vi "Load_Class_data.vi"() -> (2 "Classes":string[](array[string]), 3 "Styles and IDs":string[][](array[string]))   [LabVIEW 2025]
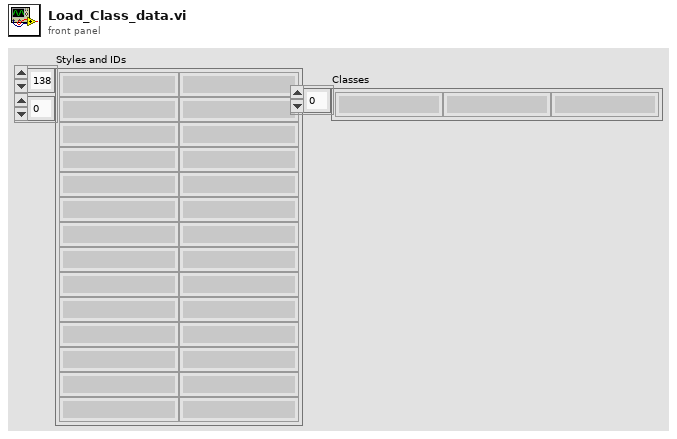
[diagram p1: front panel]
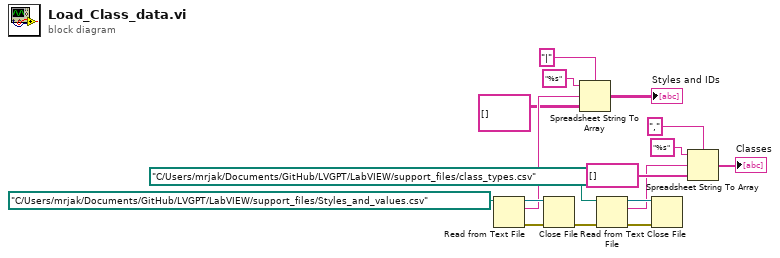
[diagram p0: block diagram]
diagram:
  n1 = Read from Text File(file (use dialog)=path "C:/Users/mrjak/Documents/GitHub/LVGPT/LabVIEW/support_files/Styles_and_values.csv") -> (refnum out=w16:refnum<file>, text=w9:string, error out=w17:errorcluster)  [unwired: 3 in, 1 out]
  n2 = Close File(refnum=w16, error in=w17) -> (error out=w13:errorcluster)  [unwired: 1 out]
  n3 = Spreadsheet String To Array(delimiter (Tab)="|", format string="%s", spreadsheet string=w9, array type (2D Dbl)=string[][] []) -> (array=→"Styles and IDs":string[][])
  n4 = Read from Text File(file (use dialog)=path "C:/Users/mrjak/Documents/GitHub/LVGPT/LabVIEW/support_files/class_types.csv", error in=w13) -> (refnum out=w15:refnum<file>, text=w3:string, error out=w14:errorcluster)  [unwired: 2 in, 1 out]
  n5 = Close File(refnum=w15, error in=w14) -> ()  [unwired: 2 out]
  n6 = Spreadsheet String To Array(delimiter (Tab)=",", format string="%s", spreadsheet string=w3, array type (2D Dbl)=string[] []) -> (array=→"Classes":string[])
